vi "Scale_X_Axis.vi"(11 "Array":refnum<vi>[](array[refnum])) -> ()   [LabVIEW 2018]
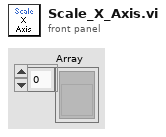
[diagram p1: front panel]
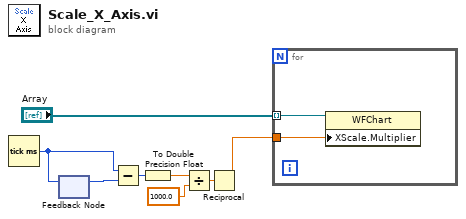
[diagram p0: block diagram]
diagram:
  n1 = Tick Count (ms)() -> (millisecond timer value=w4:u32)
  n2 = feedback #1() -> (w5:u32)  [unwired: 1 in]
  n3 = feedback-in #1(w4) -> ()
  n4 = Subtract(x=w4, y=w5) -> (x-y=w6:u32)
  n5 = To Double Precision Float(number=w6) -> (double precision float=w7:dbl)
  n6 = Divide(x=w7, y=1000.0 ("x")) -> (x/y=w2:dbl)
  n7 = Reciprocal(x=w2) -> (1/x=w8:dbl)
  n8 = for {
    tunnel: "Array" -> [w10] mode=indexing
    tunnel: w8 -> [w9]
    n9 = property class="WFChart"(reference=w10, "XScale.Multiplier"=w9) -> ()  [unwired: 1 in, 2 out]
  }
